vi "Init.vi"(8 "error in":errorcluster, 11 "Thermometer FPGA Base CFG in":refnum<class "Thermometer FPGA Base CFG.lvclass">) -> (0 "error out":errorcluster, 3 "Thermometer FPGA Base CFG out":refnum<class "Thermometer FPGA Base CFG.lvclass">)   [LabVIEW 2023, in "Thermometer FPGA Base CFG.lvclass"]
uses:
  Thermometer FPGA Base CFG.lvclass
  Thermometer FPGA Base CFG.lvclass/Thermometer FPGA Base CFG.ctl
panel:
  out "FPGA Ident":string
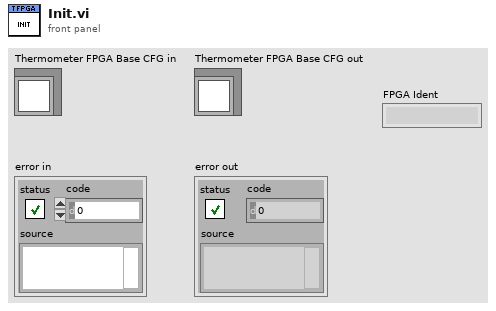
[diagram p1: front panel]
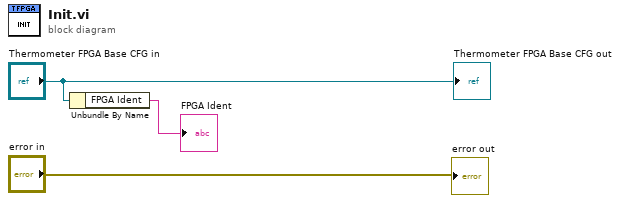
[diagram p0: block diagram]
diagram:
  n1 = Unbundle By Name("Thermometer FPGA Base CFG in") -> ("FPGA Ident"=→"FPGA Ident":string)
  "error out" <- "error in"
  "Thermometer FPGA Base CFG out" <- "Thermometer FPGA Base CFG in"
